vi "Global RefNums.vi"() -> ()   [LabVIEW 2014]
panel:
  in  "Encoder For Test":string="Test Encoder"
  in  "NavX":string="NavX"
  in  "Joystick Driver":string="Joystick Driver"
  in  "Joystick Operator":string="Joystick Operator"
  in  "Angle Resolver BR":string="Angle Resolver BR"
  in  "Angle Resolver BL":string="Angle Resolver BL"
  in  "Angle Resolver FR":string="Angle Resolver FR"
  in  "Angle Resolver FL":string="Angle Resolver FL"
  in  "Steer BR":string="Steer BR"
  in  "Steer BL":string="Steer BL"
  in  "Steer FR":string="Steer FR"
  in  "Steer FL":string="Steer FL"
  in  "Drive BR":string="Drive BR"
  in  "Drive BL":string="Drive BL"
  in  "Drive FR":string="Drive FR"
  in  "Drive FL":string="Drive FL"
  # "Actuators"
  # "Sensors"
  # "Drive"
  # "Joystick"
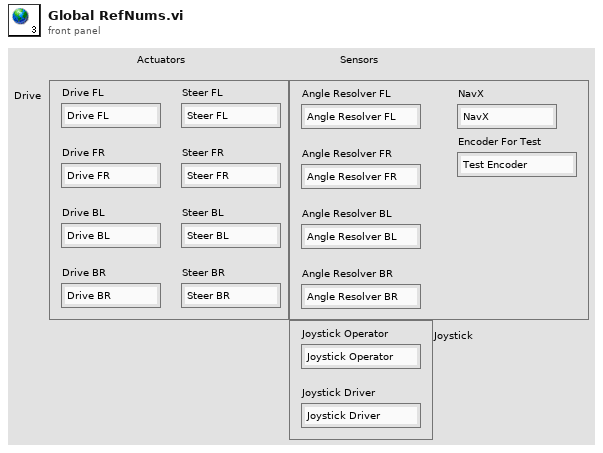
[diagram p1: front panel]
diagram:
